vi "Read ADC Response.vi"(8 "error in (no error)":errorcluster, 11 "Simulado in":refnum<class "Simulado.lvclass">) -> (0 "error out":errorcluster, 2 "Buffer":string, 3 "Simulado out":refnum<class "Simulado.lvclass">)   [LabVIEW 2020, in "Simulado.lvclass"]
doc: "Método heredado del padre con un override"
uses:
  Simulado.lvclass
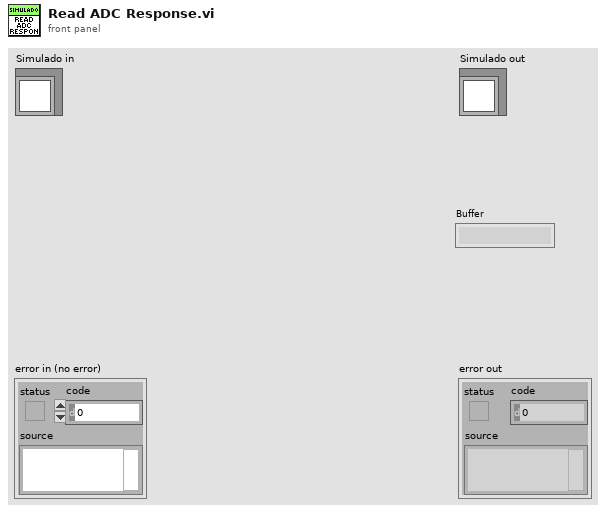
[diagram p1: front panel]
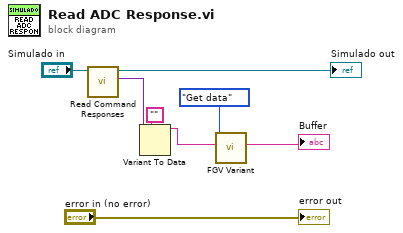
[diagram p0: block diagram]
diagram:
  n1 = call-dynamic "Read Command Responses.vi"("Simulado in"="Simulado in") -> ("Command Responses"=w3:variant, "Simulado out"=→"Simulado out":refnum<class "Simulado.lvclass">)  [unwired: 8 in, 1 out]
  n2 = Variant To Data(type="", Variant=w3) -> (data=w1:string)  [unwired: 1 in, 1 out]
  n3 = call "FGV Variant.vi"("Command"=w1, "Functions"=enum16{"Reset data", "Set data", "Get data"}."Get data") -> ("Response retrieved"=→"Buffer":string)  [unwired: 8 in, 1 out]
  "error out" <- "error in (no error)"
